vi "BooleanOps.vi"() -> ()   [LabVIEW 2019]
panel:
  out "Result":bool
  in  "b":bool
  in  "a":bool
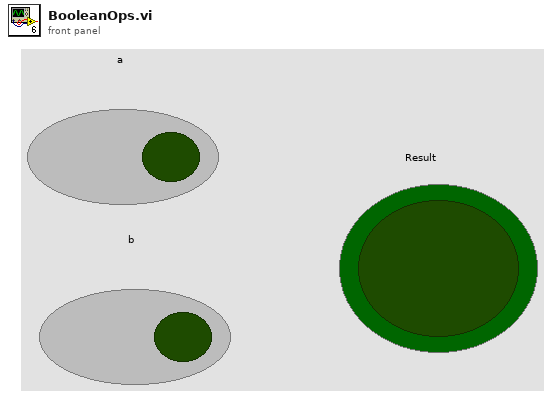
[diagram p1: front panel]
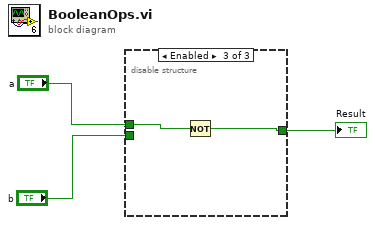
[diagram p0: block diagram]
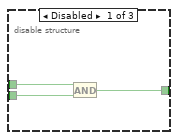
[diagram p2: hidden frame]
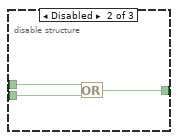
[diagram p3: hidden frame]
diagram:
  n1 = disable-structure shown="Enabled" {
    disable-tunnel: "a" -> [w6 w9 w11]
    disable-tunnel: "b" -> [w5 w8 _]
    disable-tunnel: [w4 w7 w10] -> w1
    frame Disabled {
      n2 = And(x=w6, y=w5) -> (x .and. y?=w4:bool)
    }
    frame Disabled {
      n3 = Or(x=w9, y=w8) -> (x .or. y?=w7:bool)
    }
    frame Enabled {
      n4 = Not(x=w11) -> (.not. x?=w10:bool)
    }
  }
  "Result" <- w1
